vi "Playback (fetching).vi"() -> ()   [LabVIEW 2013]
doc: "This VI reads records of data from the logging table in the LabVIEW.mdb database. \n\nThe table is opened with a static cursor pointing to the first record in the table. The DB Tools Move To Next/Previous Record VIs are used to navigate through the records when the Next and Previous buttons are pressed. The data is retrieved using the DB Tools Fetch Element Data VI and the arrays are converted from variants to LabVIEW arrays."
uses:
  Auxilliary.llb/DB Tools Cursor Type.ctl
  Connection.llb/DB Tools Open Connec (Path).vi
  Connection.llb/Conn Execute.vi
  Recordset.llb/Rec Destroy - Connection.vi
  Recordset.llb/Rec Move To Previous Record (R).vi
  Recordset.llb/Rec Get Recordset Properties (R).vi
  Recordset.llb/Rec Move To Next Record (R).vi
  Recordset.llb/Rec Fetch Binary Data (R).vi
  Recordset.llb/Rec Fetch Double Data (R).vi
  _DB Variant To Data/Database Variant To Data.xnode
  NI_Database_API_64.lvlib
panel:
  out "record number":i32
  out "Core Measuments":dbl[][](graph)
  in  "previous record":bool
  in  "next record":bool
  in  "stop":bool
  out "min temperature value":dbl format="%.2f"
  out "max temperature value":dbl format="%.2f"
  out "min pressure value":dbl format="%.2f"
  out "max pressure value":dbl format="%.2f"
  out "Core Temperature":dbl[](graph)
  out "Core Pressure":dbl[](graph)
  # "INSTRUCTIONS:\n\nRun the VI to retrieve data written by the Logging Example VI.\nOnce the VI begins, it displays the first record in the table. You can navigate the recordset using the previous record and next record buttons."
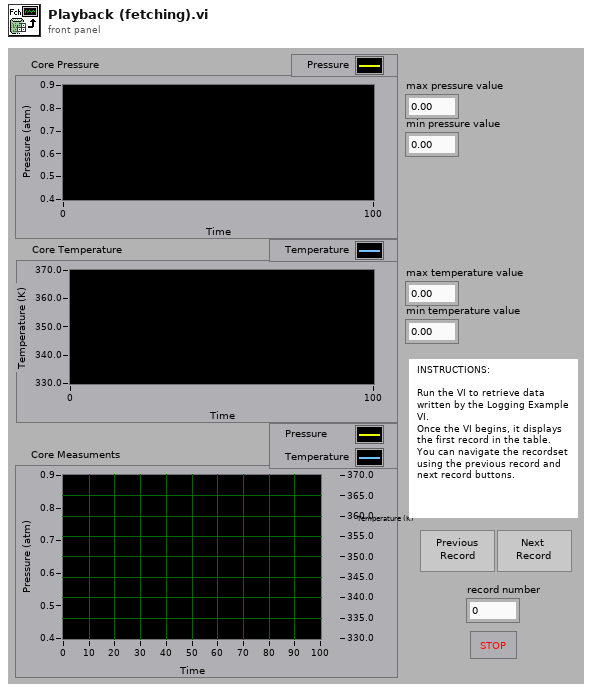
[diagram p1: front panel]
types:
  T1 = typedef "NI_Database_API_64.lvlib/DB Tools Cursor Type.ctl" = enum16{"forward-only", "keyset", "dynamic", "static"}
  T2 = typedef "NI_Database_API_64.lvlib/Conn ObjectReference.ctl" = refnum<k1>
  T3 = typedef "NI_Database_API_64.lvlib/Rec ObjectReference.ctl" = refnum<k1>
  T4 = typedef "NI_Database_API_64.lvlib/Rec Properties.ctl" = cluster{"column count":i32, "record index":i32, "record count":i32, "bof?":bool, "eof?":bool, "cursor type":T1, "cache size":i32, "state":enum16{"closed", "open"}}
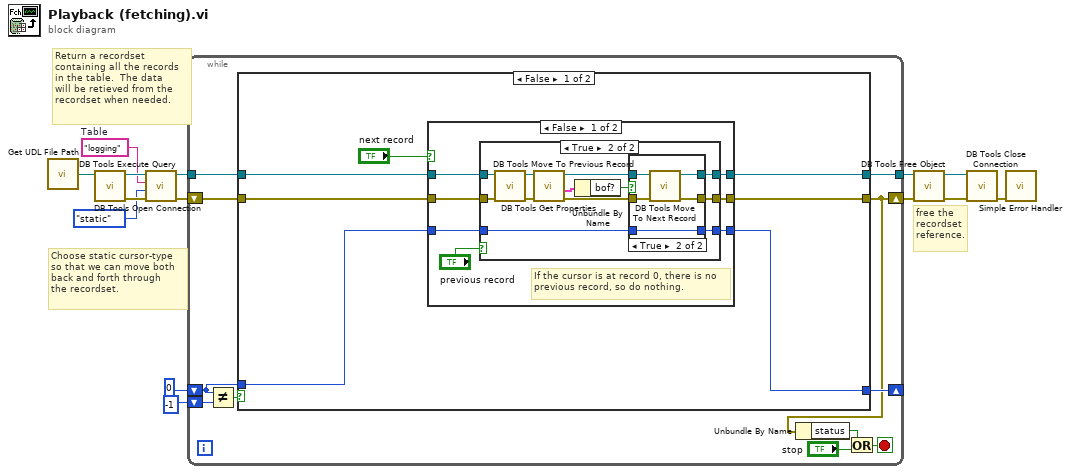
[diagram p0: block diagram]
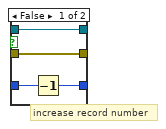
[diagram p3: hidden frame]
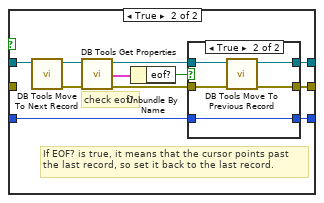
[diagram p4: hidden frame]
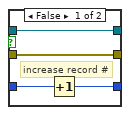
[diagram p5: hidden frame]
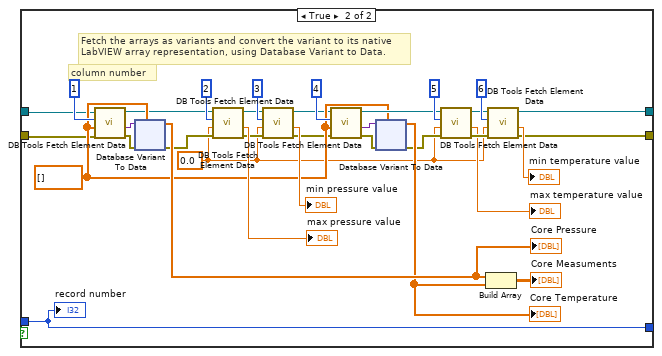
[diagram p6: hidden frame]
diagram:
  w10 = "logging"  # Table
  # "free the \nrecordset\nreference."
  # "Return a recordset \ncontaining all the records \nin the table.  The data \nwill be retieved from the \nrecordset when needed."
  # "Choose static cursor-type\nso that we can move both\nback and forth through \nthe recordset."
  n1 = call "Get UDL File Path.vi"() -> ("UDL file path"=w1:path)  [unwired: 1 in]
  n2 = call-poly "DB Tools Open Connection.vi"("connection information"=w1) -> ("error out"=w12:errorcluster, "connection reference"=w11:T2)  [unwired: 7 in]
  n3 = call-poly "DB Tools Execute Query.vi"("error in (no error)"=w12, "cursor type"=DB_Tools_Cursor_Type."static", "SQL query"=w10, "connection reference"=w11) -> ("error out"=w8:errorcluster, "recordset reference"=w9:T3)  [unwired: 4 in]
  n4 = while {
    tunnel: w9 -> [w17]
    shift-right: [w22] -> _
    shift-left: 0 -> [w23]
    shift-left: -1 -> [w25]
    shift-right: [w15] -> w5
    shift-left: w8 -> [w21]
    tunnel: [w16] -> w6
    stop <- w20 stop-if-true
    n5 = Not Equal?(x=w23, y=w25) -> (x != y?=w24:bool)
    n6 = case shown="False" w24 {
      tunnel: w23 -> [w31 w86]
      tunnel: [w30 w86] -> w22
      tunnel: w21 -> [w28 w84]
      tunnel: w17 -> [w29 w85]
      tunnel: [w27 w89] -> w15
      tunnel: [w26 w90] -> w16
      frame False {
        n7 = case shown="False" "next record" {
          tunnel: w31 -> [w39 w70]
          tunnel: [w38 w69] -> w30
          tunnel: w29 -> [w35 w65]
          tunnel: w28 -> [w34 _]
          tunnel: [w36 w68] -> w27
          tunnel: [w33 w64] -> w26
          frame False {
            # "If the cursor is at record 0, there is no \nprevious record, so do nothing."
            n8 = case shown="True" "previous record" {
              tunnel: w39 -> [w42 w46]
              tunnel: [w42 w44] -> w38
              tunnel: w34 -> [w41 w53]
              tunnel: w35 -> [w40 w54]
              tunnel: [w41 w47] -> w36
              tunnel: [w40 w43] -> w33
              frame False {
              }
              frame True {
                n9 = call-poly "DB Tools Move To Previous Record.vi"("error in (no error)"=w53, "recordset reference"=w54) -> ("error out"=w52:errorcluster, "recordset reference out"=w51:T3)  [unwired: 8 in]
                n10 = call-poly "DB Tools Get Properties.vi"("error in (no error)"=w52, "recordset reference"=w51) -> ("error out"=w49:errorcluster, "recordset properties"=w50:T4, "recordset reference out"=w48:T3)  [unwired: 3 in]
                n11 = Unbundle By Name(w50) -> ("bof?"=w45:bool)
                n12 = case shown="True" w45 {
                  tunnel: w48 -> [w55 w63]
                  tunnel: w49 -> [w56 w62]
                  tunnel: w46 -> [w58 w61]
                  tunnel: [w57 w61] -> w44
                  tunnel: [w56 w60] -> w47
                  tunnel: [w55 w59] -> w43
                  frame False {
                    # "increase record number"
                    n13 = Decrement(x=w58) -> (x-1=w57:i32)
                  }
                  frame True {
                    n14 = call-poly "DB Tools Move To Next Record.vi"("error in (no error)"=w62, "recordset reference"=w63) -> ("error out"=w60:errorcluster, "recordset reference out"=w59:T3)  [unwired: 8 in]
                  }
                }
              }
            }
          }
          frame True {
            # "If EOF? is true, it means that the cursor points past \nthe last record, so set it back to the last record."
            # "check eof?"
            n15 = call-poly "DB Tools Move To Next Record.vi"("recordset reference"=w65) -> ("error out"=w67:errorcluster, "recordset reference out"=w66:T3)  [unwired: 9 in]
            n16 = call-poly "DB Tools Get Properties.vi"("error in (no error)"=w67, "recordset reference"=w66) -> ("error out"=w71:errorcluster, "recordset properties"=w74:T4, "recordset reference out"=w72:T3)  [unwired: 3 in]
            n17 = Unbundle By Name(w74) -> ("eof?"=w73:bool)
            n18 = case shown="True" w73 {
              tunnel: w72 -> [w75 w83]
              tunnel: w71 -> [w76 w82]
              tunnel: w70 -> [w78 w81]
              tunnel: [w77 w81] -> w69
              tunnel: [w76 w80] -> w68
              tunnel: [w75 w79] -> w64
              frame False {
                # "increase record #"
                n19 = Increment(x=w78) -> (x+1=w77:i32)
              }
              frame True {
                n20 = call-poly "DB Tools Move To Previous Record.vi"("error in (no error)"=w82, "recordset reference"=w83) -> ("error out"=w80:errorcluster, "recordset reference out"=w79:T3)  [unwired: 8 in]
              }
            }
          }
        }
      }
      frame True {
        w87 = 0.0
        w96 = dbl[] [] ("Array Constant")
        # "column number"
        # "Fetch the arrays as variants and convert the variant to its native\nLabVIEW array representation, using Database Variant to Data."
        n21 = call-poly "DB Tools Fetch Element Data.vi"("error in (no error)"=w84, "type"=w96, "column index"=1 ("Index"), "recordset reference"=w85) -> ("error out"=w111:errorcluster, "data"=w112:variant, "recordset reference out"=w95:T3)  [unwired: 3 in]
        n22 = xnode "Database Variant To Data"("database variant"=w112, "error in"=w111, "type"=w96) -> ("data"=w116:dbl[], "error out"=w113:errorcluster)
        "Core Pressure" <- w116
        n23 = call-poly "DB Tools Fetch Element Data.vi"("error in (no error)"=w113, "type"=w87, "column index"=2 ("Index"), "recordset reference"=w95) -> ("error out"=w93:errorcluster, "data"=→"max pressure value":dbl, "recordset reference out"=w94:T3)  [unwired: 3 in]
        n24 = call-poly "DB Tools Fetch Element Data.vi"("error in (no error)"=w93, "type"=w87, "column index"=3 ("Index"), "recordset reference"=w94) -> ("error out"=w91:errorcluster, "data"=→"min pressure value":dbl, "recordset reference out"=w92:T3)  [unwired: 3 in]
        n25 = call-poly "DB Tools Fetch Element Data.vi"("error in (no error)"=w91, "type"=w96, "column index"=4 ("Index"), "recordset reference"=w92) -> ("error out"=w104:errorcluster, "data"=w105:variant, "recordset reference out"=w98:T3)  [unwired: 3 in]
        n26 = xnode "Database Variant To Data"("database variant"=w105, "error in"=w104, "type"=w96) -> ("data"=w106:dbl[], "error out"=w88:errorcluster)
        "Core Temperature" <- w106
        n27 = call-poly "DB Tools Fetch Element Data.vi"("error in (no error)"=w88, "type"=w87, "column index"=5 ("Index"), "recordset reference"=w98) -> ("error out"=w114:errorcluster, "data"=→"max temperature value":dbl, "recordset reference out"=w97:T3)  [unwired: 3 in]
        n28 = Build Array(w116, w106) -> (→"Core Measuments":dbl[][])
        n29 = call-poly "DB Tools Fetch Element Data.vi"("error in (no error)"=w114, "type"=w87, "column index"=6 ("Index"), "recordset reference"=w97) -> ("error out"=w89:errorcluster, "data"=→"min temperature value":dbl, "recordset reference out"=w90:T3)  [unwired: 3 in]
        "record number" <- w86
      }
    }
    n30 = Unbundle By Name(w15) -> ("status"=w18:bool)
    n31 = Or(x=w18, y="stop") -> (x .or. y?=w20:bool)
  }
  n32 = call-poly "DB Tools Free Object.vi"("error in (no error)"=w5, "recordset reference"=w6) -> ("error out"=w4:errorcluster, "connection reference"=w3:T2)  [unwired: 8 in]
  n33 = call "DB Tools Close Connection.vi"("error in (no error)"=w4, "connection reference"=w3) -> ("error out"=w2:errorcluster)  [unwired: 5 in]
  n34 = call <vilib>:"Simple Error Handler.vi"("error in (no error)"=w2) -> ()  [unwired: 4 in, 5 out]
